vi "Pack welcome byte.vi"(3 "error in":errorcluster, 4 "Serialisation":T1, 5 "Length (octets)":u8 format="%x") -> (0 "error out":errorcluster, 2 "Bytes":u8[](array[numeric]))   [LabVIEW 2020, in "wamplv.lvlib" / "RawSocket TCP Handler.lvclass"]
uses:
  RawSocket TCP Handler.lvclass
  WAMP Client/API/TypeDefs/Serialisation.ctl
  <vilib>/Utility/error.llb/Error Cluster From Error Code.vi
  <vilib>/ErrorRing/Error Ring.xnode
  RawSocket TCP Handler.lvclass/RawSocket TCP Handler.ctl
  WAMP Client/WAMP Client.lvclass
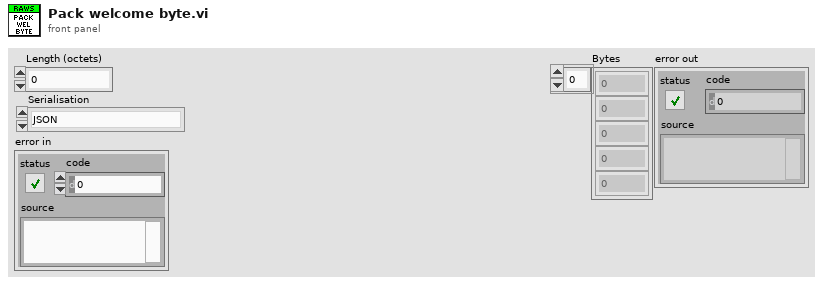
[diagram p1: front panel]
types:
  T1 = typedef "wamplv.lvlib/WAMP Client.lvclass/Serialisation.ctl" = enum16{"JSON", "MessagePack"}
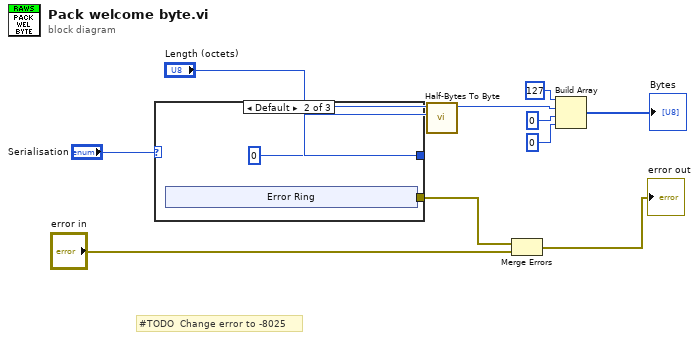
[diagram p0: block diagram]
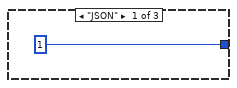
[diagram p2: hidden frame]
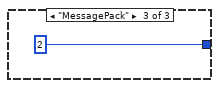
[diagram p3: hidden frame]
diagram:
  # "#TODO  Change error to -8025"
  n1 = case shown="Default" "Serialisation" {
    tunnel: [u8 1 ("Lower Half-byte") u8 0 ("Lower Half-byte") u8 2 ("Lower Half-byte")] -> w4
    tunnel: [_ w13 _] -> w2
    frame "JSON" {
    }
    frame Default {
      n2 = xnode "Error Ring"() -> ("error out"=w13:errorcluster)
    }
    frame "MessagePack" {
    }
  }
  n3 = call "Half-Bytes To Byte.vi"("Lower Half-byte"=w4, "Upper Half-Byte"="Length (octets)") -> ("Byte"=w7:u8)  [unwired: 7 in]
  n4 = Merge Errors(w2, "error in") -> (→"error out":errorcluster)
  n5 = Build Array(u8 127, w7, u8 0 ("element"), u8 0 ("element")) -> (→"Bytes":u8[])
